vi "Calculate Protection Value.vi"(4 "Length":u32, 5 "Payload Length":u32, 6 "Offset":u32, 7 "Frame ID":u32, 8 "error in (no error)":errorcluster, 9 "Overrides":dbl[](array[numeric]), 10 "Frame.Data in":dbl[](array[numeric]), 11 "Protection Configuration in":T1 {"CRC Channels"."Data Type" items=["Signed", "Unsigned", "IEEE Float"]}) -> (0 "error out":errorcluster, 1 "Protection Value":dbl, 2 "Frame.Data out":dbl[](array[numeric]), 3 "Protection Configuration out":T1 {"CRC Channels"."Data Type" items=["Signed", "Unsigned", "IEEE Float"]})   [LabVIEW 2023, in "Protection and Counter Support Engine.lvlib"]
uses:
  Protection and Counter Support Engine.lvlib
  Types/RT Protection Configuration.ctl
  Shared/Types/Protection Type.ctl
  Shared/Types/XNET Signal Configuration.ctl
  <vilib>/xnet/xnet.llb/XNET Convert (Signal to Frame Raw).vi
  LP_CRC/LP_CRC.lvlib
  Shared/Protection and Counter Support Shared.lvlib
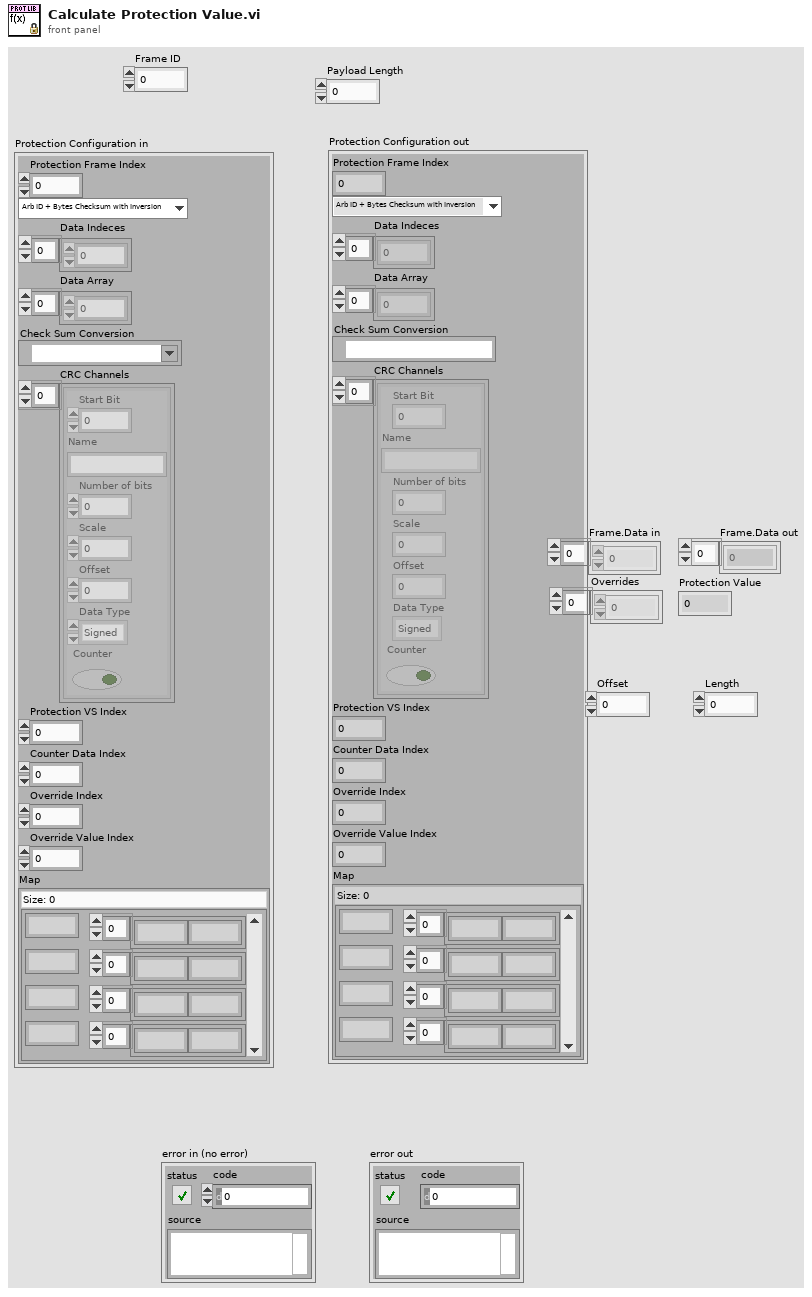
[diagram p1: front panel]
types:
  T1 = typedef "Protection and Counter Support Engine.lvlib/RT Protection Configuration.ctl" = cluster{"Protection Frame Index":i32, "Protection Type":T2, "Data Indeces":i32[], "Data Array":dbl[], "Check Sum Conversion":refnum<k21>, "CRC Channels":T3[], "Protection VS Index":i32, "Counter Data Index":i32, "Override Index":i32, "Override Value Index":i32, "Map":map{i32, u8[]}}
  T2 = typedef "Protection and Counter Support Shared.lvlib/Protection Type.ctl" = enum16{"Arb ID + Bytes Checksum with Inversion", "Arb ID + Bytes CRC with Inversion", "Reversed Raw Signal Checksum with Inversion", "Concatenated Two's Compliment", "LP_CRC8", "LP_Checksum", "LP_CRC8_MRS"}
  T3 = typedef "Protection and Counter Support Shared.lvlib/XNET Signal Configuration.ctl" = cluster{"Start Bit":i32, "Name":string, "Number of bits":i32, "Scale":dbl, "Offset":dbl, "Data Type":u32, "Counter":bool}
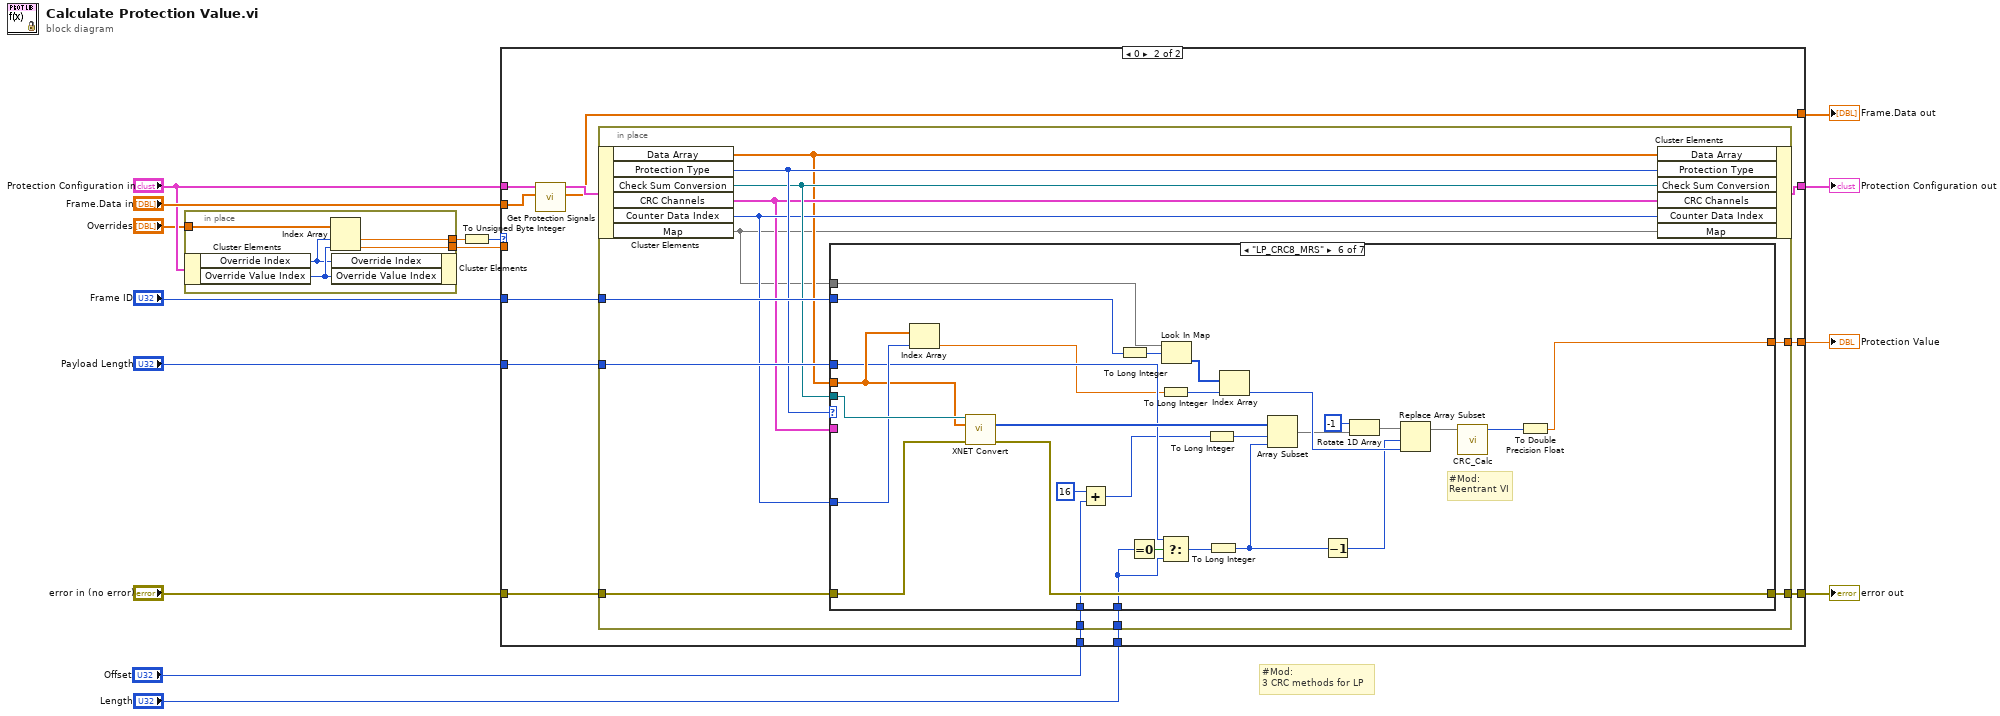
[diagram p0: block diagram]
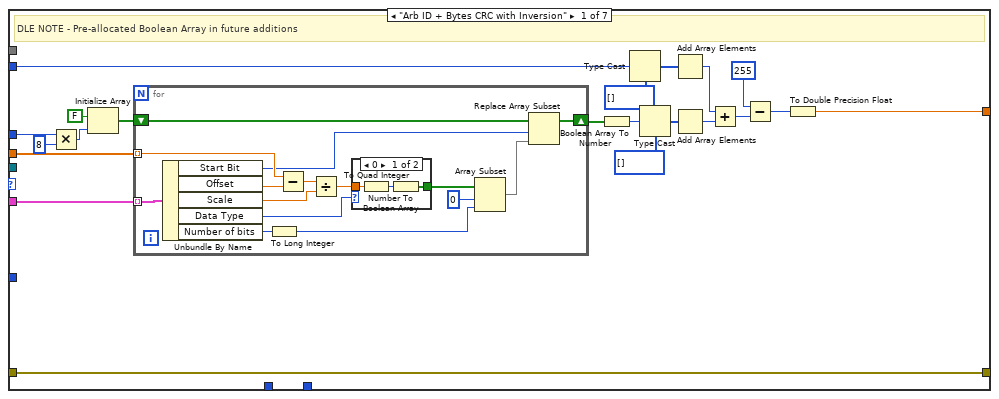
[diagram p3: hidden frame]
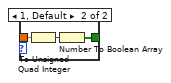
[diagram p4: hidden frame]
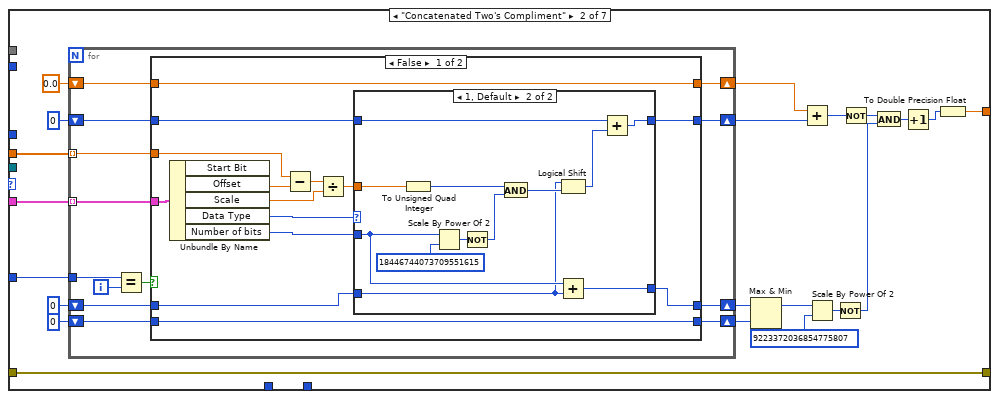
[diagram p5: hidden frame]
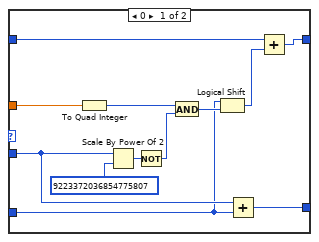
[diagram p6: hidden frame]
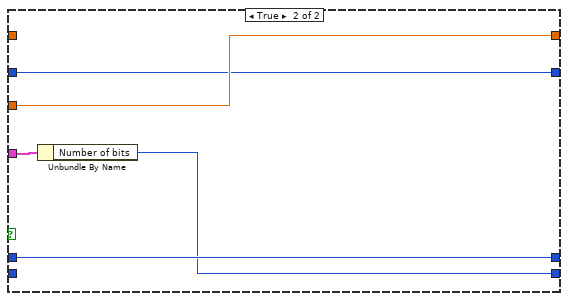
[diagram p7: hidden frame]
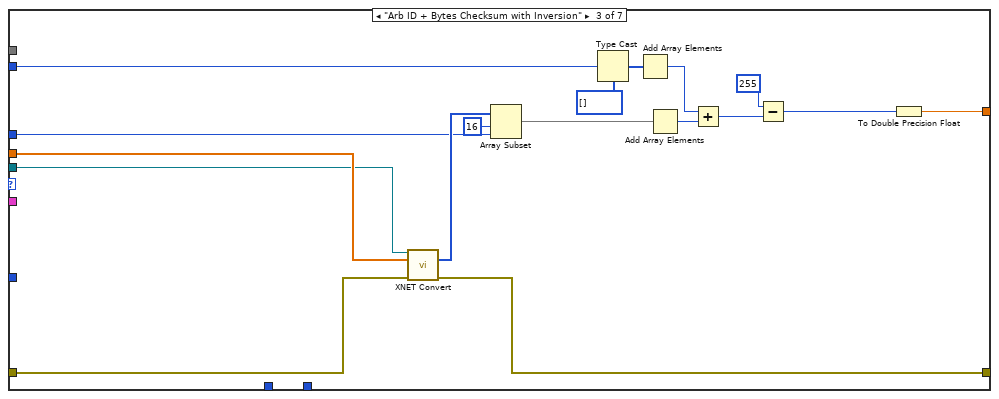
[diagram p8: hidden frame]
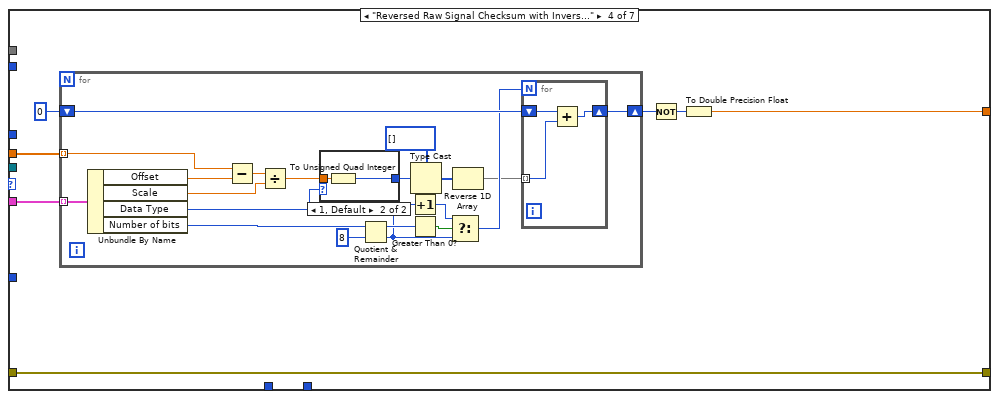
[diagram p9: hidden frame]
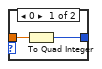
[diagram p10: hidden frame]
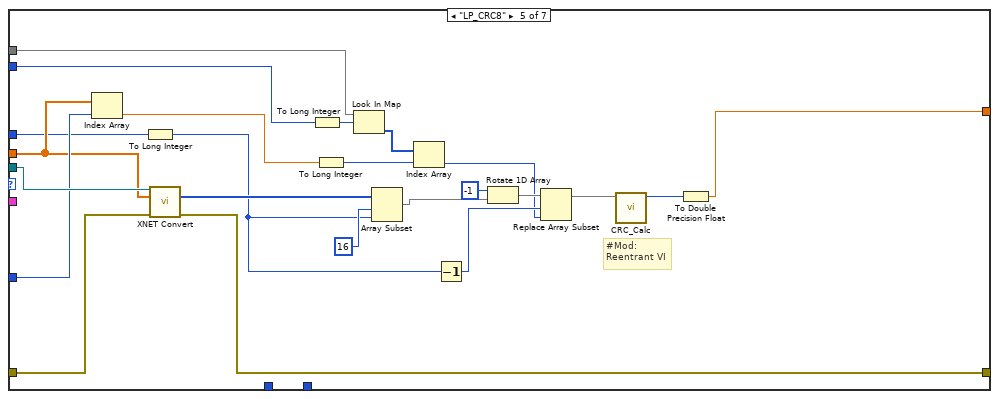
[diagram p11: hidden frame]
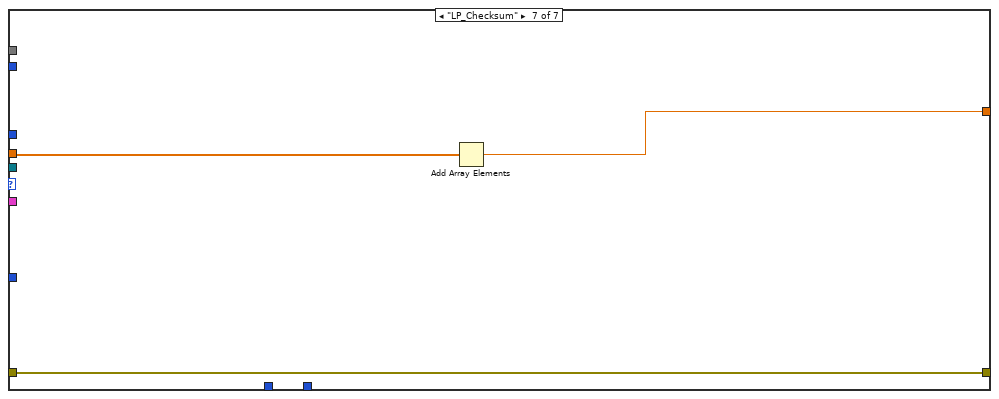
[diagram p12: hidden frame]
diagram:
  # "#Mod:\n3 CRC methods for LP"
  n1 = in-place {
    in-place-border: "Overrides" -> [w20]
    in-place-border: [w17] -> w5
    in-place-border: [w16] -> w3
    n2 = in-place-cluster #1("Protection Configuration in") -> ("Override Index"=w18:i32, "Override Value Index"=w19:i32)
    n3 = Index Array(array=w20, index #1=w18, index #2=w19) -> (element #1=w17:dbl, element #2=w16:dbl)
    n4 = in-place-cluster #1("Override Index"=w18, "Override Value Index"=w19) -> ()  [unwired: 1 out]
  }
  n5 = To Unsigned Byte Integer(number=w5) -> (unsigned 8bit integer=w4:u8)
  n6 = case shown="0" w4 {
    tunnel: "Payload Length" -> [_ w36]
    tunnel: "error in (no error)" -> [w21 w35]
    tunnel: "Frame ID" -> [_ w34]
    tunnel: [w24 w32] -> w12
    tunnel: "Frame.Data in" -> [w22 w31]
    tunnel: [w23 w30] -> w10
    tunnel: [w22 w29] -> w9
    tunnel: [w21 w28] -> w8
    tunnel: "Protection Configuration in" -> [w23 w27]
    tunnel: w3 -> [w24 _]
    tunnel: "Offset" -> [_ w26]
    tunnel: "Length" -> [_ w25]
    frame Default {
    }
    frame 0 {
      n7 = call "Get Protection Signals.vi"("Frame.Data in"=w31, "Protection Configuration"=w27) -> ("Frame.Data out"=w29:dbl[], "Protection Configuration out"=w33:T1)  [unwired: 8 in]
      n8 = in-place {
        in-place-border: w34 -> [w49]
        in-place-border: w35 -> [w48]
        in-place-border: w36 -> [w47]
        in-place-border: [w46] -> w28
        in-place-border: [w45] -> w32
        in-place-border: w26 -> [w39]
        in-place-border: w25 -> [w38]
        n9 = in-place-cluster #2(w33) -> ("Data Array"=w40:dbl[], "Protection Type"=w44:T2, "Check Sum Conversion"=w43:refnum<k21>, "CRC Channels"=w41:T3[], "Counter Data Index"=w42:i32, "Map"=w37:map{i32, u8[]})
        n10 = case shown="\"LP_CRC8_MRS\"" w44 {
          tunnel: w49 -> [w68 _ w183 _ w230 w250 _]
          tunnel: [w50 w111 w169 w186 w233 w263 w273] -> w45
          tunnel: w48 -> [w59 w112 w177 w187 w241 w270 w272]
          tunnel: [w59 w112 w176 w187 w238 w267 w272] -> w46
          tunnel: w41 -> [w57 w94 _ w190 _ _ _]
          tunnel: w40 -> [w58 w93 w173 w189 w236 w265 w274]
          tunnel: w43 -> [_ _ w172 _ w242 w271 _]
          tunnel: w47 -> [w53 _ w170 _ w225 w259 _]
          tunnel: w42 -> [_ w99 _ _ w237 w266 _]
          tunnel: w39 -> [_ _ _ _ _ w261 _]
          tunnel: w38 -> [_ _ _ _ _ w258 _]
          tunnel: w37 -> [_ _ _ _ w232 w257 _]
          frame "Arb ID + Bytes CRC with Inversion" {
            # "DLE NOTE - Pre-allocated Boolean Array in future additions"
            n11 = Multiply(x=w53, y=u32 8) -> (x*y=w52:u32)
            n12 = Initialize Array(FALSE, w52) -> (w56:bool[])
            n13 = for {
              tunnel: w57 -> [w85] mode=indexing
              shift-right: [w76] -> w62
              shift-left: w56 -> [w78]
              tunnel: w58 -> [w75] mode=indexing
              n14 = Unbundle By Name(w85) -> ("Start Bit"=w72:i32, "Offset"=w84:dbl, "Scale"=w82:dbl, "Data Type"=w74:u32, "Number of bits"=w80:i32)
              n15 = To Long Integer(number=w80) -> (32bit integer=w71:i32)
              n16 = Subtract(x=w75, y=w84) -> (x-y=w83:dbl)
              n17 = Divide(x=w83, y=w82) -> (x/y=w81:dbl)
              n18 = case shown="0" w74 {
                tunnel: w81 -> [w88 w91]
                tunnel: [w86 w89] -> w73
                frame 0 {
                  n19 = To Quad Integer(1:w88) -> (0:w87:i64)
                  n20 = Number To Boolean Array(number=w87) -> (Boolean array=w86:bool[])
                }
                frame 1, Default {
                  n21 = To Unsigned Quad Integer(1:w91) -> (0:w90:u64)
                  n22 = Number To Boolean Array(number=w90) -> (Boolean array=w89:bool[])
                }
              }
              n23 = Array Subset(array=w73, index=0, length=w71) -> (w77:bool[])
              n24 = Replace Array Subset(array=w78, new element=w77, index=w72) -> (w76:bool[])
            }
            n25 = Boolean Array To Number(Boolean array=w62) -> (number=w61:u64)
            n26 = Type Cast(type=u8[] [], x=w68) -> (*(type *) &x=w67:u8[])
            n27 = Type Cast(type=u8[] [], x=w61) -> (*(type *) &x=w54:u8[])
            n28 = Add Array Elements(numeric array=w67) -> (sum=w66:u8)
            n29 = Add Array Elements(numeric array=w54) -> (sum=w70:u8)
            n30 = Add(x=w66, y=w70) -> (x+y=w65:u8)
            n31 = Subtract(x=u8 255, y=w65) -> (x-y=w63:u8)
            n32 = To Double Precision Float(number=w63) -> (double precision float=w50:dbl)
          }
          frame "Concatenated Two's Compliment" {
            n33 = for {
              tunnel: w94 -> [w125] mode=indexing
              shift-right: [w120] -> w108
              shift-left: i64 0 -> [w123]
              tunnel: w93 -> [w124] mode=indexing
              shift-right: [w122] -> w103
              shift-left: i64 0 -> [w121]
              tunnel: w99 -> [w119]
              shift-right: [w114] -> w96
              shift-left: 0.0 -> [w116]
              shift-right: [w113] -> w95
              shift-left: i64 0 -> [w115]
              i -> [w118]
              n34 = Equal?(x=w119, y=w118) -> (x = y?=w117:bool)
              n35 = case shown="False" w117 {
                tunnel: w125 -> [w139 w168]
                tunnel: w124 -> [w134 w167]
                tunnel: w123 -> [w131 w166]
                tunnel: [w130 w165] -> w122
                tunnel: w121 -> [w129 w165]
                tunnel: [w128 w166] -> w120
                tunnel: w116 -> [w126 _]
                tunnel: w115 -> [w127 _]
                tunnel: [w126 w167] -> w114
                tunnel: [w127 w164] -> w113
                frame False {
                  n36 = Unbundle By Name(w139) -> ("Offset"=w138:dbl, "Scale"=w136:dbl, "Data Type"=w133:u32, "Number of bits"=w132:i32)  [unwired: 1 out]
                  n37 = Subtract(x=w134, y=w138) -> (x-y=w137:dbl)
                  n38 = Divide(x=w137, y=w136) -> (x/y=w135:dbl)
                  n39 = case shown="1, Default" w133 {
                    tunnel: w135 -> [w151 w161]
                    tunnel: w132 -> [w144 w157]
                    tunnel: w131 -> [w146 w155]
                    tunnel: [w143 w156] -> w130
                    tunnel: w129 -> [w141 w152]
                    tunnel: [w142 w153] -> w128
                    frame 0 {
                      n40 = To Quad Integer(1:w151) -> (0:w148:i64)
                      n41 = Scale By Power Of 2(n=w144, x=i64 9223372036854775807 ("n")) -> (x*2^n=w150:i64)
                      n42 = Not(x=w150) -> (.not. x?=w147:i64)
                      n43 = And(x=w148, y=w147) -> (x .and. y?=w145:i64)
                      n44 = Logical Shift(y=w141, x=w145) -> (x << y=w140:i64)
                      n45 = Add(x=w144, y=w141) -> (x+y=w143:i64)
                      n46 = Add(x=w146, y=w140) -> (x+y=w142:i64)
                    }
                    frame 1, Default {
                      n47 = To Unsigned Quad Integer(1:w161) -> (0:w160:u64)
                      n48 = Scale By Power Of 2(n=w157, x=u64 18446744073709551615 ("n")) -> (x*2^n=w163:u64)
                      n49 = Not(x=w163) -> (.not. x?=w159:u64)
                      n50 = And(x=w160, y=w159) -> (x .and. y?=w158:u64)
                      n51 = Logical Shift(y=w152, x=w158) -> (x << y=w154:u64)
                      n52 = Add(x=w157, y=w152) -> (x+y=w156:i64)
                      n53 = Add(x=w155, y=w154) -> (x+y=w153:i64)
                    }
                  }
                }
                frame True {
                  n54 = Unbundle By Name(w168) -> ("Number of bits"=w164:i32)
                }
              }
            }
            n55 = Max & Min(x=w103, y=w95) -> (max(x,y)=w92:i64)  [unwired: 1 out]
            n56 = Add(x=w96, y=w108) -> (x+y=w107:i64)
            n57 = Scale By Power Of 2(n=w92, x=i64 9223372036854775807 ("n")) -> (x*2^n=w105:i64)
            n58 = Not(x=w105) -> (.not. x?=w104:i64)
            n59 = Not(x=w107) -> (.not. x?=w102:i64)
            n60 = And(x=w102, y=w104) -> (x .and. y?=w101:i64)
            n61 = Increment(x=w101) -> (x+1=w106:i64)
            n62 = To Double Precision Float(number=w106) -> (double precision float=w111:dbl)
          }
          frame "Arb ID + Bytes Checksum with Inversion" {
            n63 = call-poly <vilib>:"XNET Convert.vi"("session in"=w172, "signal data"=w173, "error in (no error)"=w177) -> ("frame data"=w174:u8[], "error out"=w176:errorcluster)  [unwired: 10 in, 1 out]
            n64 = Array Subset(array=w174, index=16 ("length"), length=w170) -> (w171:u8[])
            n65 = Type Cast(type=u8[] [], x=w183) -> (*(type *) &x=w182:u8[])
            n66 = Add Array Elements(numeric array=w182) -> (sum=w181:u8)
            n67 = Add Array Elements(numeric array=w171) -> (sum=w185:u8)
            n68 = Add(x=w181, y=w185) -> (x+y=w180:u8)
            n69 = Subtract(x=u8 255, y=w180) -> (x-y=w178:u8)
            n70 = To Double Precision Float(number=w178) -> (double precision float=w169:dbl)
          }
          frame "Reversed Raw Signal Checksum with Inversion" {
            n71 = for {
              tunnel: w190 -> [w212] mode=indexing
              tunnel: w189 -> [w209] mode=indexing
              shift-right: [w206] -> w191
              shift-left: u8 0 -> [w207]
              n72 = Unbundle By Name(w212) -> ("Offset"=w211:dbl, "Scale"=w210:dbl, "Data Type"=w208:u32, "Number of bits"=w204:i32)
              n73 = Subtract(x=w209, y=w211) -> (x-y=w203:dbl)
              n74 = Divide(x=w203, y=w210) -> (x/y=w202:dbl)
              n75 = case shown="1, Default" w208 {
                tunnel: w202 -> [w217 w219]
                tunnel: [w216 w218] -> w205
                frame 0 {
                  n76 = To Quad Integer(1:w217) -> (0:w216:i64)
                }
                frame 1, Default {
                  n77 = To Unsigned Quad Integer(1:w219) -> (0:w218:u64)
                }
              }
              n78 = Quotient & Remainder(x=w204, y=8) -> (x-y*floor(x/y)=w199:i32, floor(x/y)=w197:i32)
              n79 = Increment(x=w197) -> (x+1=w198:i32)
              n80 = Greater Than 0?(x=w199) -> (x > 0?=w200:bool)
              n81 = Type Cast(type=u8[] [], x=w205) -> (*(type *) &x=w194:u8[])
              n82 = Select(t=w198, s=w200, f=w197) -> (s? t:f=w196:i32)
              n83 = Reverse 1D Array(array=w194) -> (reversed array=w193:u8[])
              n84 = for {
                N: w196 -> [_]
                tunnel: w193 -> [w214] mode=indexing
                shift-right: [w213] -> w206
                shift-left: w207 -> [w215]
                n85 = Add(x=w215, y=w214) -> (x+y=w213:u8)
              }
            }
            n86 = Not(x=w191) -> (.not. x?=w188:u8)
            n87 = To Double Precision Float(number=w188) -> (double precision float=w186:dbl)
          }
          frame "LP_CRC8" {
            # "#Mod:\nReentrant VI"
            n88 = Index Array(array=w236, index=w237) -> (element=w221:dbl)
            n89 = To Long Integer(number=w225) -> (32bit integer=w224:i32)
            n90 = call-poly <vilib>:"XNET Convert.vi"("session in"=w242, "signal data"=w236, "error in (no error)"=w241) -> ("frame data"=w235:u8[], "error out"=w238:errorcluster)  [unwired: 10 in, 1 out]
            n91 = To Long Integer(number=w230) -> (32bit integer=w231:i32)
            n92 = To Long Integer(number=w221) -> (32bit integer=w220:i32)
            n93 = Look In Map(map=w232, key=w231) -> (value=w240:u8[])  [unwired: 1 in, 1 out]
            n94 = Array Subset(array=w235, index=16 ("length"), length=w224) -> (w227:u8[])
            n95 = Index Array(array=w240, index=w220) -> (element=w222:u8)
            n96 = Decrement(x=w224) -> (x-1=w223:i32)
            n97 = Rotate 1D Array(1:w227, 2:-1 ("n")) -> (0:w228:u8[])
            n98 = Replace Array Subset(array=w228, new element=w222, index=w223) -> (w226:u8[])
            n99 = call "CRC_Calc.vi"("Data_in"=w226) -> ("CRC"=w239:u8)  [unwired: 10 in]
            n100 = To Double Precision Float(number=w239) -> (double precision float=w233:dbl)
          }
          frame "LP_CRC8_MRS" {
            # "#Mod:\nReentrant VI"
            n101 = Index Array(array=w265, index=w266) -> (element=w245:dbl)
            n102 = call-poly <vilib>:"XNET Convert.vi"("session in"=w271, "signal data"=w265, "error in (no error)"=w270) -> ("frame data"=w264:u8[], "error out"=w267:errorcluster)  [unwired: 10 in, 1 out]
            n103 = Add(x=16 ("length"), y=w261) -> (x+y=w243:u32)
            n104 = To Long Integer(number=w250) -> (32bit integer=w251:i32)
            n105 = Equal To 0?(x=w258) -> (x = 0?=w260:bool)
            n106 = To Long Integer(number=w245) -> (32bit integer=w246:i32)
            n107 = Select(t=w259, s=w260, f=w258) -> (s? t:f=w249:u32)
            n108 = Look In Map(map=w257, key=w251) -> (value=w269:u8[])  [unwired: 1 in, 1 out]
            n109 = To Long Integer(number=w243) -> (32bit integer=w244:i32)
            n110 = To Long Integer(number=w249) -> (32bit integer=w248:i32)
            n111 = Index Array(array=w269, index=w246) -> (element=w253:u8)
            n112 = Array Subset(array=w264, index=w244, length=w248) -> (w252:u8[])
            n113 = Decrement(x=w248) -> (x-1=w247:i32)
            n114 = Rotate 1D Array(1:w252, 2:-1 ("n")) -> (0:w255:u8[])
            n115 = Replace Array Subset(array=w255, new element=w253, index=w247) -> (w254:u8[])
            n116 = call "CRC_Calc.vi"("Data_in"=w254) -> ("CRC"=w268:u8)  [unwired: 10 in]
            n117 = To Double Precision Float(number=w268) -> (double precision float=w263:dbl)
          }
          frame "LP_Checksum" {
            n118 = Add Array Elements(numeric array=w274) -> (sum=w273:dbl)
          }
        }
        n119 = in-place-cluster #2("Data Array"=w40, "Protection Type"=w44, "Check Sum Conversion"=w43, "CRC Channels"=w41, "Counter Data Index"=w42, "Map"=w37) -> (w30:T1)
      }
    }
  }
  "Protection Configuration out" <- w10
  "error out" <- w8
  "Frame.Data out" <- w9
  "Protection Value" <- w12
